vi "Create Label String.vi"(8 "error in (no error)":errorcluster, 10 "Actual Range In":T3, 11 "3D Plot.lvclass in":refnum<class "3D Plot.lvclass">) -> (0 "error out":errorcluster, 1 "Label Cluster":T1, 2 "Actual Range Out":T3, 3 "3D Plot.lvclass out":refnum<class "3D Plot.lvclass">)   [LabVIEW 2020, in "3D Plot.lvclass"]
uses:
  3D Plot.lvclass
  Range Clusters.ctl
  Tick Array Cluster.ctl
  Tick Array.ctl
  3D Plot.lvclass/3D Plot.ctl
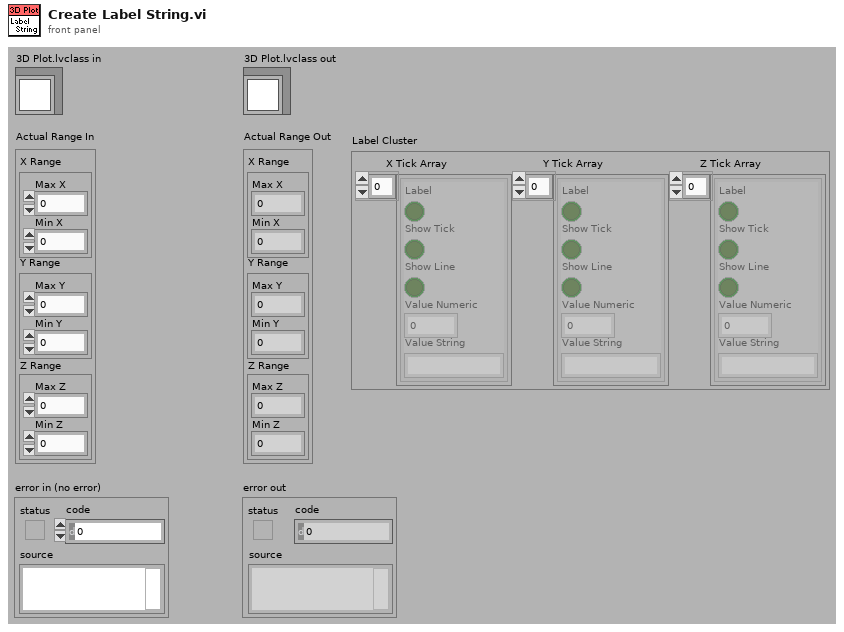
[diagram p1: front panel]
types:
  T1 = typedef "3D Plot.lvclass/Tick Array Cluster.ctl" = cluster{"X Tick Array":T2, "Y Tick Array":T2, "Z Tick Array":T2}
  T2 = typedef "3D Plot.lvclass/Tick Array.ctl" = cluster{"Label":bool, "Show Tick":bool, "Show Line":bool, "Value Numeric":sgl, "Value String":string}[]
  T3 = typedef "3D Plot.lvclass/Range Clusters.ctl" = cluster{"X Range":cluster{"Max X":sgl, "Min X":sgl}, "Y Range":cluster{"Max Y":sgl, "Min Y":sgl}, "Z Range":cluster{"Max Z":sgl, "Min Z":sgl}}
  T4 = typedef "3D Plot.lvclass/Format Property.ctl" = string[]
  T5 = typedef "3D Plot.lvclass/Value Pair Property.ctl" = T6[]
  T6 = typedef "3D Plot.lvclass/Value Pair Cluster.ctl" = cluster{"Value Pair Array":cluster{"Value":sgl, "Name":string}[], "Show Tick":bool, "Show Grid":bool, " Label Mode":enum16{"Name", "Value", "None"}}
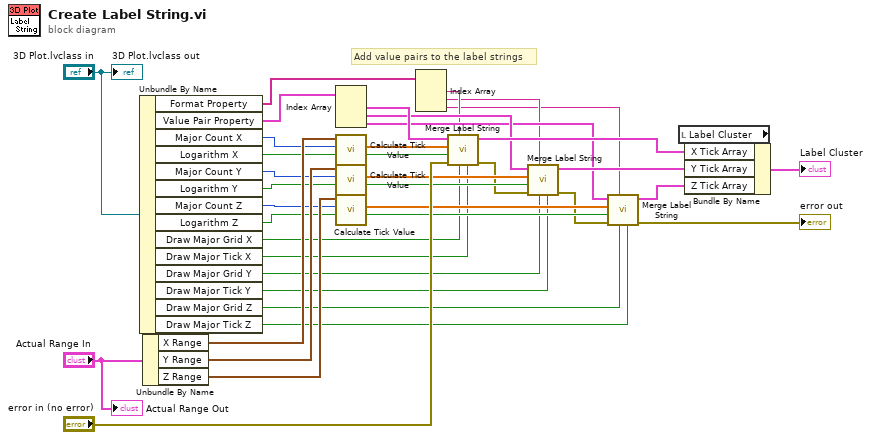
[diagram p0: block diagram]
diagram:
  # "Add value pairs to the label strings"
  n1 = Unbundle By Name("3D Plot.lvclass in") -> ("Format Property"=w14:T4, "Value Pair Property"=w18:T5, "Major Count X"=w19:u16, "Logarithm X"=w8:bool, "Major Count Y"=w7:u16, "Logarithm Y"=w6:bool, "Major Count Z"=w5:u16, "Logarithm Z"=w25:bool, "Draw Major Grid X"=w10:bool, "Draw Major Tick X"=w4:bool, "Draw Major Grid Y"=w3:bool, "Draw Major Tick Y"=w2:bool, "Draw Major Grid Z"=w1:bool, "Draw Major Tick Z"=w9:bool)
  n2 = Unbundle By Name("Actual Range In") -> ("X Range"=w35:cluster{"Max X":sgl, "Min X":sgl}, "Y Range"=w33:cluster{"Max Y":sgl, "Min Y":sgl}, "Z Range"=w34:cluster{"Max Z":sgl, "Min Z":sgl})
  n3 = Index Array(array=w18) -> (element #1=w17:T6, element #2=w16:T6, element #3=w15:T6)  [unwired: 3 in]
  n4 = call "Calculate Tick Value.vi"("Logarithm?"=w8, "Tick Count"=w19, "Axis Range"=w35) -> ("Logarithm?"=w24:bool, "Tick Value Array"=w29:sgl[])  [unwired: 1 in, 6 out]
  n5 = call "Calculate Tick Value.vi"("Logarithm?"=w6, "Tick Count"=w7, "Axis Range"=w33) -> ("Logarithm?"=w23:bool, "Tick Value Array"=w28:sgl[])  [unwired: 2 in, 5 out]
  n6 = call "Calculate Tick Value.vi"("Logarithm?"=w25, "Tick Count"=w5, "Axis Range"=w34) -> ("Logarithm?"=w22:bool, "Tick Value Array"=w27:sgl[])  [unwired: 1 in, 6 out]
  n7 = Index Array(array=w14) -> (element #1=w13:string, element #2=w12:string, element #3=w11:string)  [unwired: 3 in]
  n8 = call "Merge Label String.vi"("Draw Major Tick?"=w4, "Draw Major Grid?"=w10, "Format String"=w13, "error in (no error)"="error in (no error)", "Logarithm?"=w24, "Tick Value Array"=w29, "Value Pair Cluster"=w17) -> ("error out"=w21:errorcluster, "Tick Cluster Array"=w30:T2)  [unwired: 3 out]
  n9 = call "Merge Label String.vi"("Draw Major Tick?"=w2, "Draw Major Grid?"=w3, "Format String"=w12, "error in (no error)"=w21, "Logarithm?"=w23, "Tick Value Array"=w28, "Value Pair Cluster"=w16) -> ("error out"=w20:errorcluster, "Tick Cluster Array"=w31:T2)  [unwired: 3 out]
  n10 = call "Merge Label String.vi"("Draw Major Tick?"=w9, "Draw Major Grid?"=w1, "Format String"=w11, "error in (no error)"=w20, "Logarithm?"=w22, "Tick Value Array"=w27, "Value Pair Cluster"=w15) -> ("error out"=→"error out":errorcluster, "Tick Cluster Array"=w32:T2)  [unwired: 3 out]
  n11 = local read "Label Cluster"() -> (w26:T1)
  n12 = Bundle By Name(cluster=w26, "X Tick Array"=w30, "Y Tick Array"=w31, "Z Tick Array"=w32) -> (→"Label Cluster":T1)
  "Actual Range Out" <- "Actual Range In"
  "3D Plot.lvclass out" <- "3D Plot.lvclass in"
